vi "ThorlabsMode.vi"(8 "error in":errorcluster, 10 "Mode":u16(ring) items=["Manual"=1, "XGate"=5], 11 "VISA resource name":refnum<visa-resource-name>) -> (0 "error out":errorcluster, 3 "VISA resource name out":refnum<visa-resource-name>)   [LabVIEW 2018]
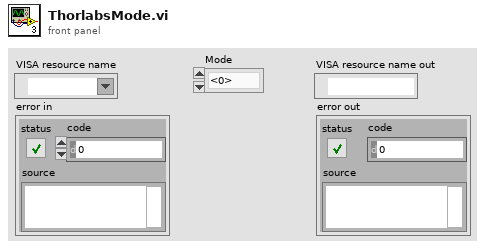
[diagram p1: front panel]
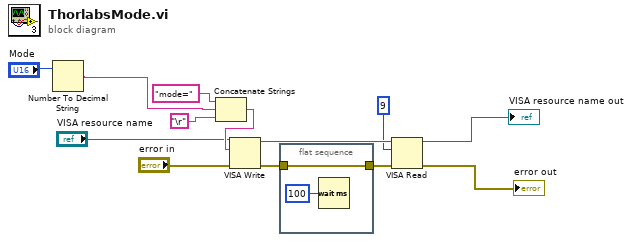
[diagram p0: block diagram]
diagram:
  n1 = Number To Decimal String(number="Mode") -> (decimal integer string=w1:string)  [unwired: 1 in]
  n2 = Concatenate Strings("mode=" ("write buffer"), w1, "\r") -> (w12:string)
  n3 = VISA Write(VISA resource name="VISA resource name", write buffer=w12, error in (no error)="error in") -> (VISA resource name out=w13:refnum<visa-resource-name>, error out=w9:errorcluster)  [unwired: 1 out]
  n4 = flat-sequence {
    tunnel: w9 -> [w14]
    tunnel: [w14] -> w8
    frame #0 {
      n5 = Wait (ms)(milliseconds to wait=u32 100) -> ()  [unwired: 1 out]
    }
  }
  n6 = VISA Read(VISA resource name=w13, byte count=u32 9, error in (no error)=w8) -> (VISA resource name out=→"VISA resource name out":refnum<visa-resource-name>, error out=→"error out":errorcluster)  [unwired: 2 out]
